vi "close underlying connection.vi"(8 "error in":errorcluster, 11 "connection in":refnum<class "TCP connection.lvclass">) -> (0 "error out":errorcluster)   [LabVIEW 2015, in "TCP connection.lvclass"]
uses:
  TCP connection.lvclass
  TCP connection.lvclass/TCP connection.ctl
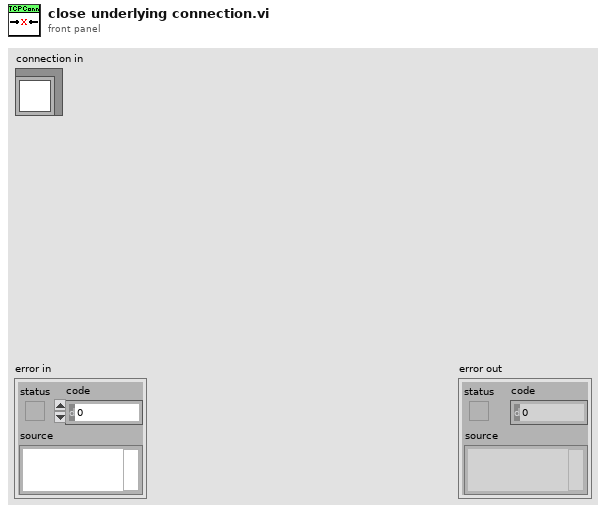
[diagram p1: front panel]
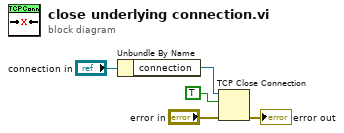
[diagram p0: block diagram]
diagram:
  n1 = Unbundle By Name("connection in") -> ("connection"=w2:refnum<k5>)
  n2 = TCP Close Connection(connection ID=w2, abort (F)=TRUE, error in (no error)="error in") -> (error out=→"error out":errorcluster)  [unwired: 1 out]
